vi "Read Filter Configuration Array.vi"(11 "Main Display in":refnum<class "Main Display.lvclass">) -> (2 "Filter Configuration Array":refnum<class "Base Filter.lvclass">[](array[class]))   [LabVIEW 2018, in "Assert API Components.lvlib" / "Assert Display.lvlib" / "Main Display.lvlib" / "Main Display.lvclass"]
uses:
  Main Display.lvclass
  Assert API Components/Filter Configurations/Base Filter.lvclass
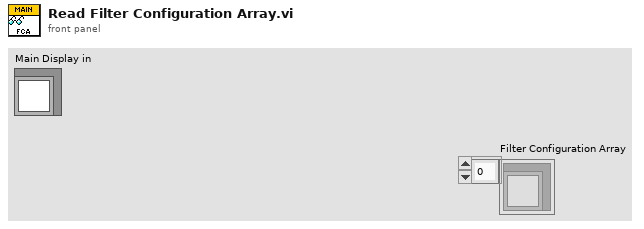
[diagram p1: front panel]
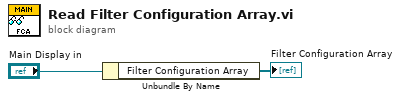
[diagram p0: block diagram]
diagram:
  n1 = Unbundle By Name("Main Display in") -> ("Filter Configuration Array"=→"Filter Configuration Array":refnum<class "Base Filter.lvclass">[])
